vi "Autosize MCListbox Row Header Column.vi"(4 "Default Width":u32=50, 6 "Whitespace Border":i16=10, 8 "error in":errorcluster, 9 "reference in":refnum<vi>) -> (0 "error out":errorcluster, 1 "reference out":refnum<vi>)   [LabVIEW 2015]
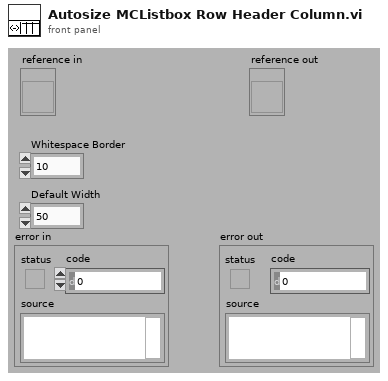
[diagram p1: front panel]
types:
  T1 = enum16{"User-specified Font", "Application Font", "System Font", "Dialog Font"}
  T2 = cluster{"Font Name:":string, "Size":i16, "Strikeout?":bool, "Italic?":bool, "Underline?":bool, "Outline?":bool, "Shadow?":bool, "Bold?":bool}
  T3 = cluster{"left":i16, "top":i16, "right":i16, "bottom":i16}
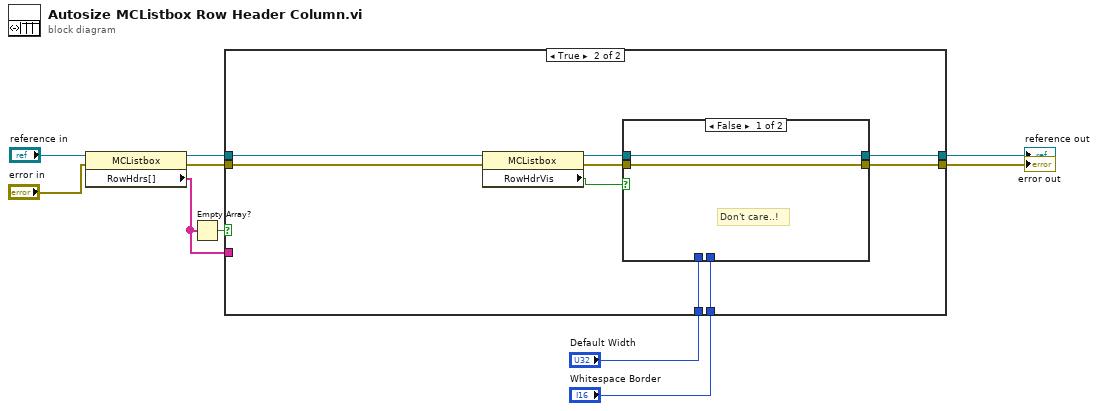
[diagram p0: block diagram]
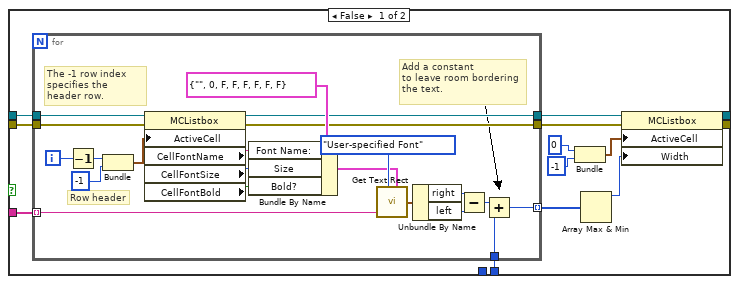
[diagram p2: hidden frame]
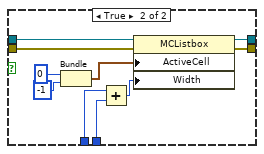
[diagram p3: hidden frame]
diagram:
  n1 = property class="MCListbox"(reference="reference in", error in="error in") -> (reference out=w5:refnum<vi>, error out=w4:errorcluster, "RowHdrs[]"=w3:string[])
  n2 = Empty Array?(array=w3) -> (empty?=w2:bool)
  n3 = case shown="True" w2 {
    tunnel: w3 -> [w16 _]
    tunnel: w5 -> [w15 w49]
    tunnel: w4 -> [w14 w47]
    tunnel: [w13 w53] -> w8
    tunnel: [w12 w52] -> w9
    tunnel: "Whitespace Border" -> [w11 w50]
    tunnel: "Default Width" -> [_ w51]
    frame False {
      n4 = for {
        tunnel: w15 -> [w44]
        tunnel: [w28] -> w23 mode=indexing
        tunnel: w14 -> [w33]
        tunnel: [w32] -> w21
        tunnel: [w31] -> w22
        tunnel: w11 -> [w26]
        tunnel: w16 -> [w24] mode=indexing
        i -> [w27]
        # "The -1 row index specifies the header row."
        # "Add a constant\nto leave room bordering the text."
        # "Row header"
        n5 = Decrement(x=w27) -> (x-1=w34:i32)
        n6 = Bundle(w34, -1) -> (w43:cluster{i32, i32})  [unwired: 1 out]
        n7 = property class="MCListbox"(reference=w44, error in=w33, "ActiveCell"=w43) -> (reference out=w31:refnum<vi>, error out=w32:errorcluster, "CellFontName"=w41:string, "CellFontSize"=w29:u32, "CellFontBold"=w40:bool)
        n8 = Bundle By Name(cluster=T2 {"Font Name:"="", "Size"=0, "Strikeout?"=FALSE, "Italic?"=FALSE, "Underline?"=FALSE, "Outline?"=FALSE, "Shadow?"=FALSE, "Bold?"=FALSE} ("[user-specified font]"), "Font Name:"=w41, "Size"=w29, "Bold?"=w40) -> (w38:T2)
        n9 = call <vilib>:"Get Text Rect.vi"("desired font(Application)"=T1."User-specified Font", "text"=w24, "[user-specified font]"=w38) -> ("rect"=w37:T3)  [unwired: 3 in, 3 out]
        n10 = Unbundle By Name(w37) -> ("right"=w36:i16, "left"=w35:i16)
        n11 = Subtract(x=w36, y=w35) -> (x-y=w30:i16)
        n12 = Add(x=w30, y=w26) -> (x+y=w28:i16)
      }
      n13 = Bundle(0, -1) -> (w19:cluster{i32, i32})  [unwired: 1 out]
      n14 = Array Max & Min(array=w23) -> (max value=w18:i16)  [unwired: 3 out]
      n15 = property class="MCListbox"(reference=w22, error in=w21, "ActiveCell"=w19, "Width"=w18) -> (reference out=w13:refnum<vi>, error out=w12:errorcluster)
    }
    frame True {
      n16 = property class="MCListbox"(reference=w49, error in=w47) -> (reference out=w48:refnum<vi>, error out=w46:errorcluster, "RowHdrVis"=w45:bool)
      n17 = case shown="False" w45 {
        tunnel: [w55 w62] -> w53
        tunnel: [w54 w61] -> w52
        tunnel: w51 -> [_ w60]
        tunnel: w50 -> [_ w59]
        tunnel: w48 -> [w55 w57]
        tunnel: w46 -> [w54 w56]
        frame False {
          # "Don't care..!"
        }
        frame True {
          n18 = Bundle(0, -1) -> (w64:cluster{i32, i32})  [unwired: 1 out]
          n19 = Add(x=w60, y=w59) -> (x+y=w58:u32)
          n20 = property class="MCListbox"(reference=w57, error in=w56, "ActiveCell"=w64, "Width"=w58) -> (reference out=w62:refnum<vi>, error out=w61:errorcluster)
        }
      }
    }
  }
  "error out" <- w9
  "reference out" <- w8
